vi "Movimiento_3Ejes(SubVi).vi"(2 "Cluster":T1={"Motion Resource 1"="Eje X", "Motion Resource 2"="Eje Y", "Motion Resource 3"="EJE Z", "Posición_1"=20.0, "Posición_2"=10.0, "Posición_3"=5.0, "Velocidad"=4.0, "Dif_1"=10.0, "Dif_2"=5.0, "Dif_3"=2.5}) -> (0 "Done":bool)   [LabVIEW 2017]
uses:
  <vilib>/Motion/Express/_s/nimc.fb.straightLineMove.startStraightLineMove.axis.modeAbsolute.0.vi
  <vilib>/Motion/BlockNode/FB.NIMotion.xnode
panel:
  out "Numeric Control 3":dbl
  out "Numeric Control 2":dbl
  out "Numeric Control":dbl
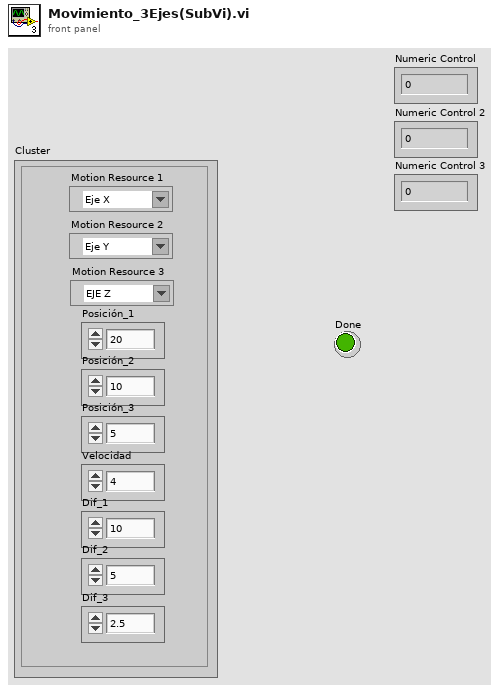
[diagram p1: front panel]
types:
  T1 = cluster{"Motion Resource 1":refnum<k21>, "Motion Resource 2":refnum<k21>, "Motion Resource 3":refnum<k21>, "Posición_1":dbl, "Posición_2":dbl, "Posición_3":dbl, "Velocidad":dbl, "Dif_1":dbl, "Dif_2":dbl, "Dif_3":dbl}
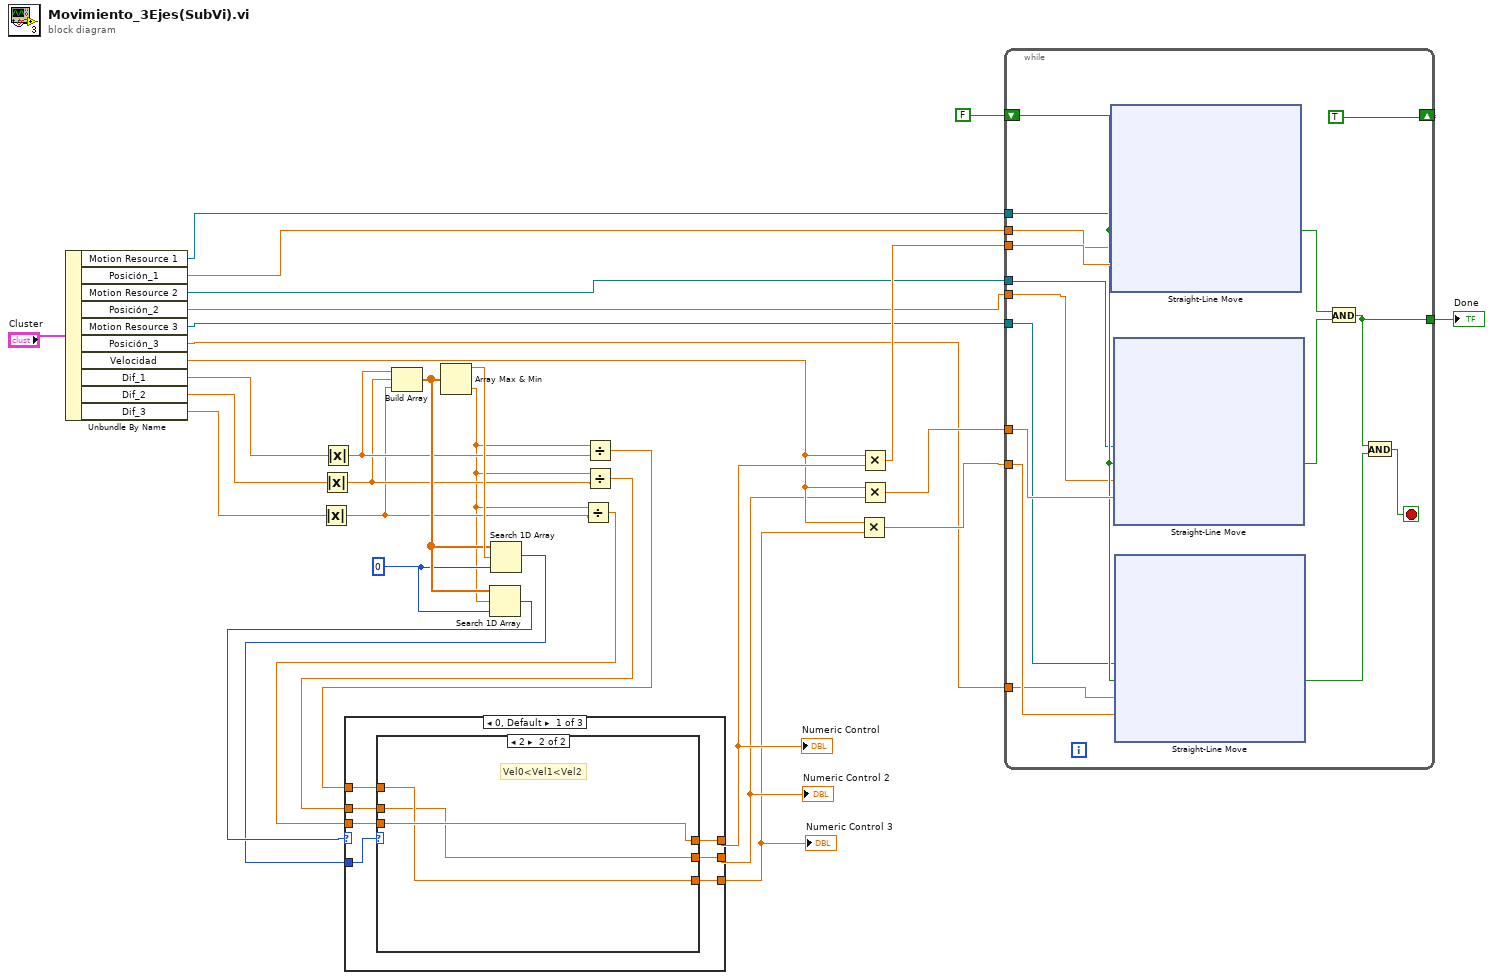
[diagram p0: block diagram]
diagram:
  w23 = 0
  n1 = Unbundle By Name("Cluster") -> ("Motion Resource 1"=w3:refnum<k21>, "Posición_1"=w8:dbl, "Motion Resource 2"=w2:refnum<k21>, "Posición_2"=w5:dbl, "Motion Resource 3"=w1:refnum<k21>, "Posición_3"=w4:dbl, "Velocidad"=w12:dbl, "Dif_1"=w28:dbl, "Dif_2"=w27:dbl, "Dif_3"=w26:dbl)
  n2 = Absolute Value(x=w26) -> (abs(x)=w18:dbl)
  n3 = Absolute Value(x=w27) -> (abs(x)=w19:dbl)
  n4 = Absolute Value(x=w28) -> (abs(x)=w20:dbl)
  n5 = Build Array(w20, w19, w18) -> (w24:dbl[])
  n6 = Array Max & Min(array=w24) -> (max value=w25:dbl, min value=w17:dbl)  [unwired: 2 out]
  n7 = Search 1D Array(1D array=w24, element=w17, start index (0)=w23) -> (index of element=w22:i32)
  n8 = Search 1D Array(1D array=w24, element=w25, start index (0)=w23) -> (index of element=w21:i32)
  n9 = Divide(x=w17, y=w18) -> (x/y=w14:dbl)
  n10 = Divide(x=w17, y=w20) -> (x/y=w16:dbl)
  n11 = Divide(x=w17, y=w19) -> (x/y=w15:dbl)
  n12 = case shown="0, Default" w22 {
    tunnel: w21 -> [w38 w45 w58]
    tunnel: w16 -> [w37 w49 w63]
    tunnel: w15 -> [w36 w51 w62]
    tunnel: w14 -> [w35 w50 w59]
    tunnel: [w34 w47 w61] -> w10
    tunnel: [w33 w46 w60] -> w11
    tunnel: [w32 w48 w64] -> w13
    frame 0, Default {
      n13 = case shown="2" w38 {
        tunnel: w37 -> [w40 w43]
        tunnel: w36 -> [w39 w42]
        tunnel: w35 -> [w41 w44]
        tunnel: [w41 w43] -> w34
        tunnel: [w40 w42] -> w33
        tunnel: [w39 w44] -> w32
        frame 1, Default {
          # "Vel0<Vel2<Vel1"
        }
        frame 2 {
          # "Vel0<Vel1<Vel2"
        }
      }
    }
    frame 1 {
      n14 = case shown="2" w45 {
        tunnel: w51 -> [w52 w56]
        tunnel: w50 -> [w54 w55]
        tunnel: w49 -> [w53 w57]
        tunnel: [w52 w57] -> w48
        tunnel: [w54 w56] -> w47
        tunnel: [w53 w55] -> w46
        frame 0, Default {
          # "Vel1<Vel2<Vel0"
        }
        frame 2 {
          # "Vel1<Vel0<Vel2"
        }
      }
    }
    frame 2 {
      n15 = case shown="1" w58 {
        tunnel: [w67 w70] -> w64
        tunnel: w63 -> [w66 w70]
        tunnel: w62 -> [w65 w69]
        tunnel: [w66 w69] -> w61
        tunnel: [w65 w68] -> w60
        tunnel: w59 -> [w67 w68]
        frame 0, Default {
          # "Vel2<Vel0<Vel0"
        }
        frame 1 {
          # "Vel2<Vel0<Vel1"
        }
      }
    }
  }
  "Numeric Control" <- w13
  "Numeric Control 2" <- w11
  "Numeric Control 3" <- w10
  n16 = Multiply(x=w12, y=w10) -> (x*y=w7:dbl)
  n17 = Multiply(x=w12, y=w13) -> (x*y=w9:dbl)
  n18 = Multiply(x=w12, y=w11) -> (x*y=w6:dbl)
  n19 = while {
    shift-right: [TRUE] -> _
    shift-left: FALSE -> [w77]
    tunnel: [w81] -> w30
    tunnel: w9 -> [w80]
    tunnel: w6 -> [w79]
    tunnel: w7 -> [w78]
    tunnel: w8 -> [w76]
    tunnel: w5 -> [w75]
    tunnel: w4 -> [w74]
    tunnel: w3 -> [w73]
    tunnel: w2 -> [w72]
    tunnel: w1 -> [w71]
    stop <- w82 stop-if-true
    n20 = xnode "Straight-Line Move"("resource"=w73, "execute"=w77, "position"=w76, "velocity"=w80) -> ("done"=w85:bool)  [unwired: 2 in, 2 out]
    n21 = xnode "Straight-Line Move"("resource"=w72, "execute"=w77, "position"=w75, "velocity"=w79) -> ("done"=w84:bool)  [unwired: 2 in, 2 out]
    n22 = xnode "Straight-Line Move"("resource"=w71, "execute"=w77, "position"=w74, "velocity"=w78) -> ("done"=w83:bool)  [unwired: 2 in, 2 out]
    n23 = And(x=w85, y=w84) -> (x .and. y?=w81:bool)
    n24 = And(x=w81, y=w83) -> (x .and. y?=w82:bool)
  }
  "Done" <- w30
